vi "reset.vi"(8 "error in (no error)":errorcluster, 11 "FgenNiPxi in":refnum<class "ArbNi.lvclass">) -> (0 "error out":errorcluster, 3 "FgenNiPxi out":refnum<class "ArbNi.lvclass">)   [LabVIEW 2023, in "ArbNi.lvclass"]
doc: "<b>Author:</b> Wolfgang\n<b>Description:</b> This method is used to reset the instrument to a default and known state."
uses:
  ArbNi.lvclass
  ArbNi.lvclass/ArbNi.ctl
  Arb.lvclass
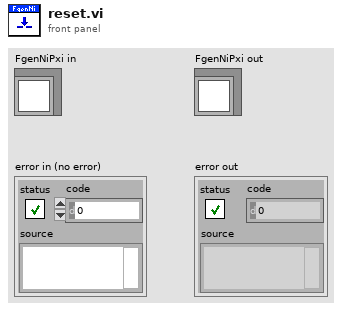
[diagram p1: front panel]
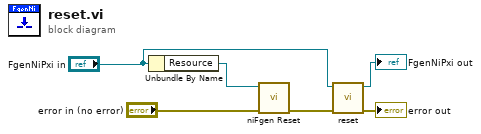
[diagram p0: block diagram]
diagram:
  n1 = Unbundle By Name("FgenNiPxi in") -> ("Resource"=w4:refnum<k15>)
  n2 = call <instrlib>:"niFgen Reset.vi"("error in (no error)"="error in (no error)", "Instrument Handle"=w4) -> ("error out"=w2:errorcluster)  [unwired: 8 in, 1 out]
  n3 = call-parent "reset.vi"("error in (no error)"=w2, "Instrument in"="FgenNiPxi in") -> ("error out"=→"error out":errorcluster, "Instrument out"=→"FgenNiPxi out":refnum<class "ArbNi.lvclass">)  [unwired: 8 in]
